vi "SeCrTs-Do State extracter.vi"(8 "error in":errorcluster, 9 "input cluster":T1={"AO config"=[], "AI config"=[], "DI config"=[], "DO config"=[], "TC config"=[], "ACC config"=[], "SG config"=[], "Strain Gauge Settings"={"poisson ratio"=0.0, "nominal gage resistance"=120.0, "gage factor"=2.0}, "Bridge Settings"={"voltage excitation value"=3.0, "voltage excitation source"=10200, "initial bridge voltage"=0.0, "lead wire resistance"=1.7, "strain configuration"=10271}, "Sample Rate"={"AI Sample Rate"=[], "AO Sample Rate"=[], "DI Sample Rate"=[], "TC Sample Rate"=[], "DO Sample Rate"=[], "SG Sample Rate"=[], "ACC Sample Rate"=[]}} {"Bridge Settings"."strain configuration" items=["Full Bridge I"=10183, "Full Bridge II"=10184, "Full Bridge III"=10185, "Half Bridge I"=10188, "Half Bridge II"=10189, "Quarter Bridge I"=10271, "Quarter Bridge II"=10272]; "Bridge Settings"."voltage excitation source" items=["Internal"=10200, "External"=10167, "None"=10230]; "ACC config"."Terminal configuration" items=["default"=-1, "RSE"=10083, "NRSE"=10078, "Differential"=10106, "Pseudodifferential"=12529]; "ACC config"."Sensitivity units" items=["mVolts/g"=12509, "Volts/g"=12510]; "TC config"."type" items=["J"=10072, "K"=10073, "N"=10077, "R"=10082, "S"=10085, "T"=10086, "B"=10047, "E"=10055]; "TC config"."units" items=["Deg C", "Deg F", "Kelvins", "Deg R", "From Custom Scale"]}, 11 "EPV ref":refnum<vi>[](array[refnum])) -> (0 "error out":errorcluster)   [LabVIEW 2022 SP3]
uses:
  Controls/SeCrTs-Config.ctl
panel:
  out "Array 2":i32[](array[numeric])
  out "Array":string[](array[string])
  in  "Names":string[](array[string])=["NC_EPV_1211", "NO_EPV_1102", "NC_EPV_1214", "NO_EPV_1207", "AC_Button", "NC_EPV_481", "NO_EPV_478R", "NO_EPV_477", "NC_EPV_56", "NO_EPV_122", "NC_EPV_61", "NC_EPV_1001", "F_EPV_1004", "F_EPV_1008", "N_EPV_1091", "NC_EPV_1217", "F_EPV_1007"]
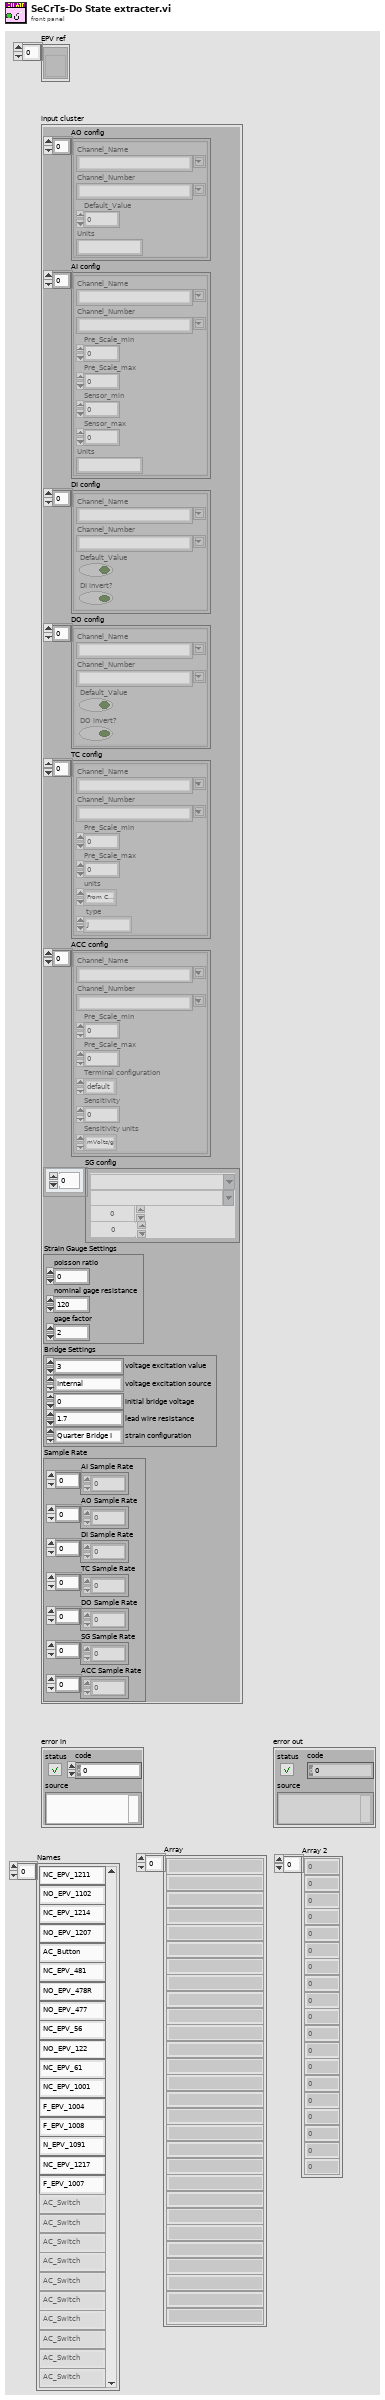
[diagram p1: front panel]
types:
  T1 = typedef "SeCrTs-Config.ctl" = cluster{"AO config":cluster{"Channel_Name":string, "Channel_Number":string, "Default_Value":dbl, "Units":string}[], "AI config":cluster{"Channel_Name":string, "Channel_Number":string, "Pre_Scale_min":dbl, "Pre_Scale_max":dbl, "Sensor_min":dbl, "Sensor_max":dbl, "Units":string}[], "DI config":cluster{"Channel_Name":string, "Channel_Number":string, "Default_Value":bool, "DI invert?":bool}[], "DO config":cluster{"Channel_Name":string, "Channel_Number":string, "Default_Value":bool, "DO invert?":bool}[], "TC config":cluster{"Channel_Name":string, "Channel_Number":string, "Pre_Scale_min":dbl, "Pre_Scale_max":dbl, "units":i32, " type":i32}[], "ACC config":cluster{"Channel_Name":string, "Channel_Number":string, "Pre_Scale_min":dbl, "Pre_Scale_max":dbl, "Terminal configuration":i32, "Sensitivity":dbl, "Sensitivity units":i32}[], "SG config":cluster{"Channel_Name":string, "Channel_Number":string, "Pre_Scale_min":dbl, "Pre_Scale_max":dbl}[], "Strain Gauge Settings":cluster{"poisson ratio":dbl, "nominal gage resistance":dbl, "gage factor":dbl}, "Bridge Settings":cluster{"voltage excitation value":dbl, "voltage excitation source":i32, "initial bridge voltage":dbl, "lead wire resistance":dbl, "strain configuration":i32}, "Sample Rate":cluster{"AI Sample Rate":dbl[], "AO Sample Rate":dbl[], "DI Sample Rate":dbl[], "TC Sample Rate":dbl[], "DO Sample Rate":dbl[], "SG Sample Rate":dbl[], "ACC Sample Rate":dbl[]}}
  T2 = cluster{"Channel_Name":string, "Channel_Number":string, "Default_Value":bool, "DO invert?":bool}[]
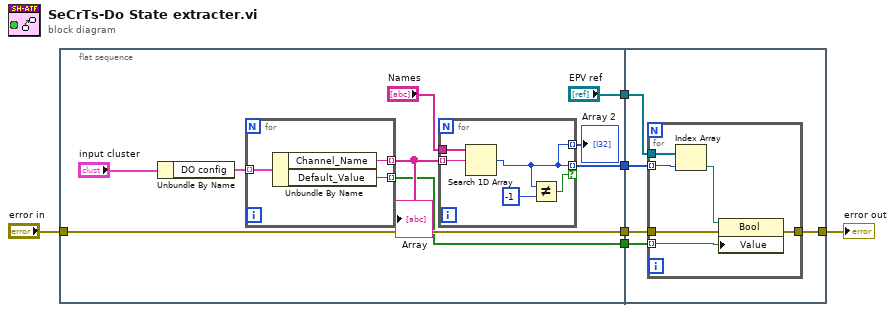
[diagram p0: block diagram]
diagram:
  n1 = flat-sequence {
    tunnel: [w12] -> w6
    tunnel: [w11] -> w5
    tunnel: "error in" -> [w11]
    tunnel: ["EPV ref"] -> w2
    tunnel: [w8] -> w1
    tunnel: w6 -> [w28]
    tunnel: w5 -> [w27]
    tunnel: [w26] -> w3
    tunnel: w2 -> [w25]
    tunnel: w1 -> [w24]
    frame #0 {
      n2 = Unbundle By Name("input cluster") -> ("DO config"=w15:T2)
      n3 = for {
        tunnel: w15 -> [w23] mode=indexing
        tunnel: [w22] -> w13 mode=indexing
        tunnel: [w21] -> w8 mode=indexing
        n4 = Unbundle By Name(w23) -> ("Channel_Name"=w22:string, "Default_Value"=w21:bool)
      }
      "Array" <- w13
      n5 = for {
        tunnel: w13 -> [w19] mode=indexing
        tunnel: [w16] -> w12 mode=indexing if=w17
        tunnel: "Names" -> [w20]
        tunnel: [w16] -> w7 mode=indexing
        n6 = Search 1D Array(1D array=w20, element=w19) -> (index of element=w16:i32)  [unwired: 1 in]
        n7 = Not Equal?(x=w16, y=-1) -> (x != y?=w17:bool)
      }
      "Array 2" <- w7
    }
    frame #1 {
      n8 = for {
        tunnel: w25 -> [w34]
        tunnel: w28 -> [w30] mode=indexing
        tunnel: w27 -> [w33]
        tunnel: [w32] -> w26
        tunnel: w24 -> [w29] mode=indexing
        n9 = Index Array(array=w34, index=w30) -> (element=w31:refnum<vi>)
        n10 = property class="Bool"(reference=w31, error in=w33, "Value"=w29) -> (error out=w32:errorcluster)  [unwired: 1 out]
      }
    }
  }
  "error out" <- w3
